vi "LinearSystemLoop_SngJntArm_Pack_Ctrl.vi"(6 "Max Ctrl Out V":dbl=12.0, 7 "Ang Model Std Dev Rad":dbl=0.5, 8 "Vel Ctrl Tol Rad/Sec":dbl=0.8, 9 "Ang Ctrl Tol Rad":dbl=0.06, 10 "Ang Meas Std Dev Rad":dbl=0.02, 11 "Vel Model Std Dev Rad/Sec":dbl=20.0) -> (3 "LinearSystemLoop_SngJntArm_Ctrl_Params":T1={"Ang Model Std Dev Rad"=0.0, "Ang Meas Std Dev Rad"=0.0, "Ang Ctrl Tol Rad"=0.0, "Max Ctrl Out V"=0.0, "Vel Model Std Dev Rad/Sec"=0.8, "Vel Ctrl Tol Rad/Sec"=0.02})   [LabVIEW 2019, in "Trajectory_Library.lvlib"]
doc: "The single jointed arm linear system definition is:\n - States\n - angle position (Rad)\n - Inputs:\n - motor voltage\n - Outputs:\n - angle position (rad)"
uses:
  Trajectory_Library.lvlib
  TypeDef/LINEAR_SYSTEM_LOOP_SNGJNTARM_CTRL_PARAMS.ctl
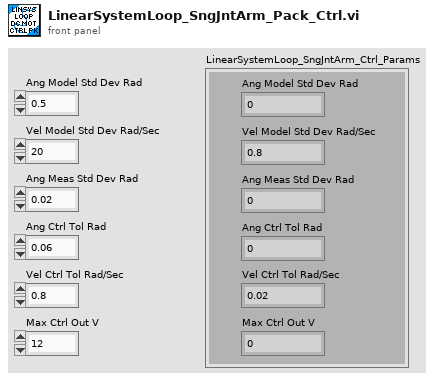
[diagram p1: front panel]
types:
  T1 = typedef "Trajectory_Library.lvlib/LINEAR_SYSTEM_LOOP_SNGJNTARM_CTRL_PARAMS.ctl" = cluster{"Ang Model Std Dev Rad":dbl, "Ang Meas Std Dev Rad":dbl, "Ang Ctrl Tol Rad":dbl, "Max Ctrl Out V":dbl, "Vel Model Std Dev Rad/Sec":dbl, "Vel Ctrl Tol Rad/Sec":dbl}
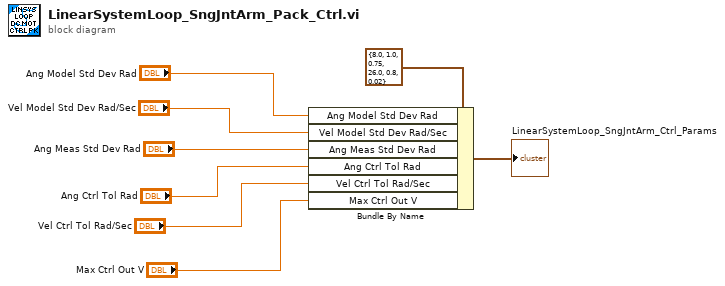
[diagram p0: block diagram]
diagram:
  n1 = Bundle By Name(cluster=T1 {"Ang Model Std Dev Rad"=8.0, "Ang Meas Std Dev Rad"=1.0, "Ang Ctrl Tol Rad"=0.75, "Max Ctrl Out V"=26.0, "Vel Model Std Dev Rad/Sec"=0.8, "Vel Ctrl Tol Rad/Sec"=0.02} ("DCMotorSim_Model _Params"), "Ang Model Std Dev Rad"="Ang Model Std Dev Rad", "Vel Model Std Dev Rad/Sec"="Vel Model Std Dev Rad/Sec", "Ang Meas Std Dev Rad"="Ang Meas Std Dev Rad", "Ang Ctrl Tol Rad"="Ang Ctrl Tol Rad", "Vel Ctrl Tol Rad/Sec"="Vel Ctrl Tol Rad/Sec", "Max Ctrl Out V"="Max Ctrl Out V") -> (→"LinearSystemLoop_SngJntArm_Ctrl_Params":T1)
